vi "solar_app SOLARini Read (BOOL).vi"(5 "Write If Not Found? (T)":bool=TRUE, 6 "Comment (Create only)":string, 7 "Section (\"\"=solar)":string, 9 "Default Value (BOOL)":bool, 10 "Key":string) -> (1 "Value (BOOL) out":bool, 2 "Found?":bool)   [LabVIEW 2018]
doc: "This reads a boolean configuration key from the solar.ini configuration file."
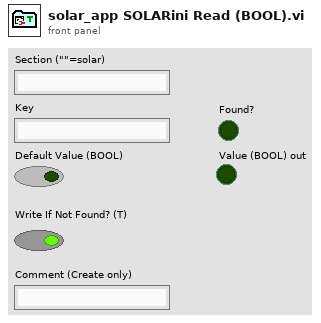
[diagram p1: front panel]
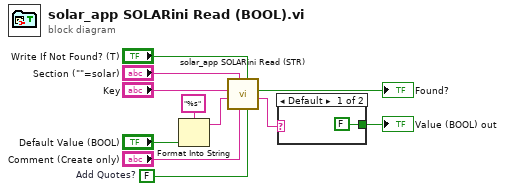
[diagram p0: block diagram]
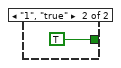
[diagram p2: hidden frame]
diagram:
  w6 = FALSE  # Add Quotes?
  n1 = Format Into String(format string="%s", "Default Value (BOOL)") -> (resulting string=w7:string)  [unwired: 2 in, 1 out]
  n2 = call "solar_app SOLARini Read (STR).vi"("Add Quotes? (T)"=w6, "Write If Not Found? (T)"="Write If Not Found? (T)", "Comment (Create only)"="Comment (Create only)", "Section (\"\"=solar)"="Section (\"\"=solar)", "Default Value (STR)"=w7, "Key"="Key") -> ("Value (STR) out"=w4:string, "Found?"=→"Found?":bool)  [unwired: 4 in]
  n3 = case shown="Default" w4 {
    tunnel: [FALSE TRUE] -> w3
    frame Default {
    }
    frame "1", "true" {
    }
  }
  "Value (BOOL) out" <- w3
